vi "Get Info.vi"(8 "error in (no error)":errorcluster, 11 "AInterestAccount in":refnum<class "AInterestAccount.lvclass">) -> (0 "error out":errorcluster, 2 "Account Information":T1, 3 "AInterestAccount out":refnum<class "AInterestAccount.lvclass">)   [LabVIEW 2020, in "AInterestAccount.lvclass"]
uses:
  AInterestAccount.lvclass
  Account Information STYP.ctl
  AInterestAccount.lvclass/AInterestAccount.ctl
  AAccount/AAccount.lvclass
  IInfoable/IInfoable.lvclass
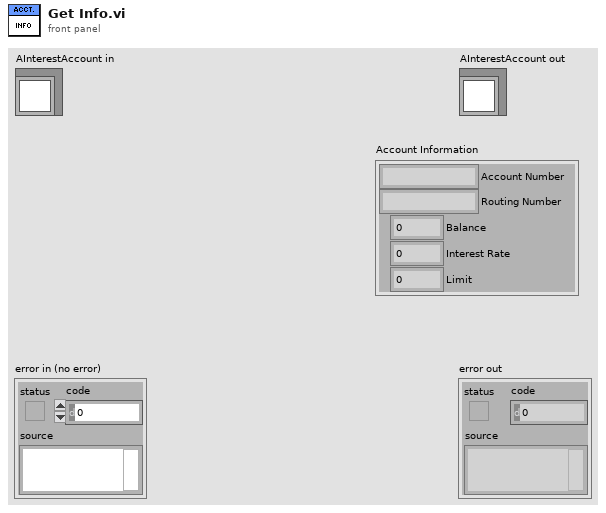
[diagram p1: front panel]
types:
  T1 = typedef "IInfoable.lvclass/Account Information STYP.ctl" = cluster{"Account Number":string, "Routing Number":string, "Balance":dbl, "Interest Rate":dbl, "Limit":dbl}
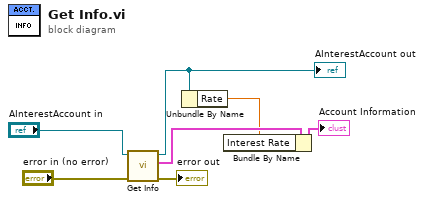
[diagram p0: block diagram]
diagram:
  n1 = call-parent "Get Info.vi"("error in (no error)"="error in (no error)", "AAccount in"="AInterestAccount in") -> ("error out"=→"error out":errorcluster, "Account Information"=w6:T1, "AAccount out"=w2:refnum<class "AInterestAccount.lvclass">)  [unwired: 7 in]
  "AInterestAccount out" <- w2
  n2 = Unbundle By Name(w2) -> ("Rate"=w1:dbl)
  n3 = Bundle By Name(cluster=w6, "Interest Rate"=w1) -> (→"Account Information":T1)
